vi "Routine.vi"(11 "TEMPLATE Event in":refnum<class "TEMPLATE Event.lvclass">) -> (3 "TEMPLATE Event out":refnum<class "TEMPLATE Event.lvclass">)   [LabVIEW 2021, in "_Template.lvlib" / "Templates.lvlib" / "TEMPLATE Event.lvlib" / "TEMPLATE Event.lvclass"]
uses:
  TEMPLATE Event.lvclass
  <vilib>/Nathan Davis/jettl/jettl/Event/Event.lvclass
  <vilib>/Nathan Davis/jettl/jettl/Msg Strategy/Msg Strategy.lvclass
  C:/Program Files/National Instruments/LabVIEW 2021/vi.lib/Nathan Davis/jettl/jettl/jettl/jettl.lvclass
panel:
  # "Note the VI Properties have been modified for typical UI window settings.\n\nThis panel operates as a normal user interface.\nClick the Panel Close? for the default implemention to occur: executing the Teardown method."
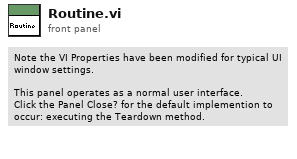
[diagram p1: front panel]
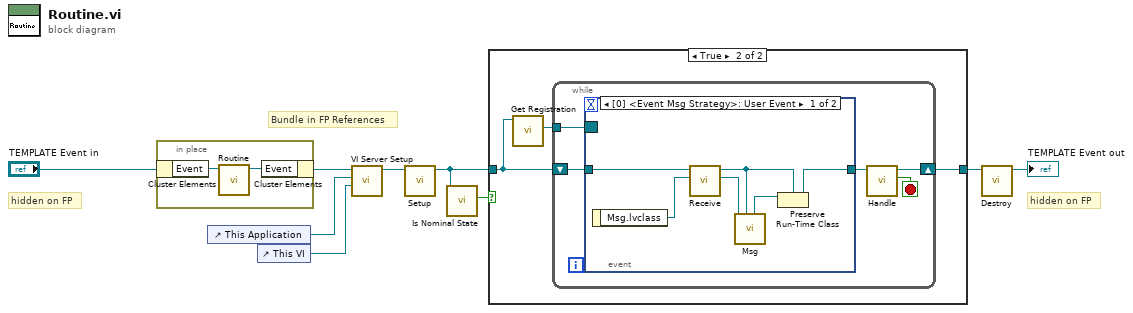
[diagram p0: block diagram]
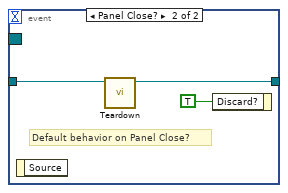
[diagram p3: hidden frame]
diagram:
  # "Bundle in FP References"
  # "hidden on FP"
  # "hidden on FP"
  n1 = in-place {
    n2 = in-place-cluster #1("TEMPLATE Event in") -> ("Event"=w11:refnum<class "Event.lvclass">)
    n3 = call-dynamic "Routine.vi"("jettl in"=w11) -> ("jettl out"=w10:refnum<class "Event.lvclass">)  [unwired: 10 in]
    n4 = in-place-cluster #1("Event"=w10) -> (w4:refnum<class "TEMPLATE Event.lvclass">)
  }
  n5 = control-ref of="This Application"() -> (w2:refnum<vi>)
  n6 = control-ref of="This VI"() -> (w1:refnum<vi>)
  n7 = call-dynamic "VI Server Setup.vi"("This VI"=w1, "This Application"=w2, "TEMPLATE Event in"=w4) -> ("TEMPLATE Event out"=w3:refnum<class "TEMPLATE Event.lvclass">)  [unwired: 8 in]
  n8 = call-dynamic "Setup.vi"("TEMPLATE Event in"=w3) -> ("TEMPLATE Event out"=w6:refnum<class "TEMPLATE Event.lvclass">)  [unwired: 10 in]
  n9 = call-dynamic "Is Nominal State.vi"("TEMPLATE Event in"=w6) -> ("Is Nominal State?"=w5:bool)  [unwired: 10 in]
  n10 = case shown="True" w5 {
    tunnel: w6 -> [w12 w15]
    tunnel: [w12 w13] -> w8
    frame False {
    }
    frame True {
      n11 = call-dynamic "Get Registration.vi"("TEMPLATE Event in"=w15) -> ("Registration"=w14:refnum<event-registration>)  [unwired: 10 in]
      n12 = while {
        shift-right: [w17] -> w13
        shift-left: w15 -> [w19]
        tunnel: w14 -> [w20]
        stop <- w16 stop-if-true
        n13 = event shown="[0] <Event Msg Strategy>: User Event" {
          selector: w20 -> [_ _]
          dyn-events: _ -> [_ _]
          timeout: _ -> [_ _]
          tunnel: w19 -> [w24 w28]
          tunnel: [w26 w27] -> w18
          event User Event {
            n14 = event-data() -> ("Msg.lvclass"=w21:refnum<class "Msg Strategy.lvclass">)  [unwired: 1 in]
            n15 = call-dynamic "Receive.vi"("Msg Strategy in"=w21, "TEMPLATE Event in"=w24) -> ("Msg Strategy out"=w22:refnum<class "Msg Strategy.lvclass">, "TEMPLATE Event out"=w23:refnum<class "TEMPLATE Event.lvclass">)  [unwired: 8 in]
            n16 = call-dynamic "Msg.vi"("jettl in"=w23, "Msg Strategy in"=w22) -> ("jettl out"=w25:refnum<class "jettl.lvclass">)  [unwired: 9 in]
            n17 = Preserve Run-Time Class(object in=w25, 2:w23) -> (object out=w26:refnum<class "TEMPLATE Event.lvclass">)  [unwired: 1 in, 1 out]
          }
          event Panel Close? {
            # "Default behavior on Panel Close?"
            n18 = event-data() -> ()  [unwired: 1 in, 1 out]
            n19 = call-dynamic "Teardown.vi"("TEMPLATE Event in"=w28) -> ("TEMPLATE Event out"=w27:refnum<class "TEMPLATE Event.lvclass">)  [unwired: 10 in]
            n20 = event-data("Discard?"=TRUE) -> ()  [unwired: 1 in, 1 out]
          }
        }
        n21 = call-dynamic "Handle.vi"("TEMPLATE Event in"=w18) -> ("Destroy?"=w16:bool, "TEMPLATE Event out"=w17:refnum<class "TEMPLATE Event.lvclass">)  [unwired: 9 in]
      }
    }
  }
  n22 = call-dynamic "Destroy.vi"("TEMPLATE Event in"=w8) -> ("TEMPLATE Event out"=→"TEMPLATE Event out":refnum<class "TEMPLATE Event.lvclass">)  [unwired: 10 in]
